vi "Convert FCS to PT3.vi"() -> ()   [LabVIEW 2012]
uses:
  Online acquisition/Online correlation/TTTR_data_headers/BINHDR_P.ctl
  Online acquisition/Online correlation/TTTR_data_headers/BOARDHDR.ctl
  Online acquisition/Online correlation/TTTR_data_headers/RtChan.ctl
  Online acquisition/Online correlation/TTTR_data_headers/TTTRHDR_P.ctl
  Online acquisition/Online correlation/TTTR_data_headers/TXTHDR.ctl
panel:
  out "Progress":dbl(slide) scale=0.0..100.0
  in  "Tab PH300":enum32{"PicoHarp 300 pt3 headers"}(tab)
  out "BINHDR_P":T1
  out "BOARDHDR":T2={"HardwareIdent[16]"="PicoHarp 300", "HardwareVersion[8]"="2.0", "HardwareSerial"=1006456, "SyncDivider"=8, "CFDZeroCross0"=10, "CFDLevel0"=200, "CFDZeroCross1"=10, "CFDLevel1"=200, "Resolution"=0.016, "RouterModelCode"=0, "RouterEnabled"=1, "RtChan"=[{"InputType"=1, "InputLevel"=-325, "InputEdge"=0, "CFDPresent"=0, "CFDLevel"=0, "CFDZeroCross"=0}, {"InputType"=1, "InputLevel"=-325, "InputEdge"=0, "CFDPresent"=0, "CFDLevel"=0, "CFDZeroCross"=0}, {"InputType"=2, "InputLevel"=760, "InputEdge"=1, "CFDPresent"=0, "CFDLevel"=1, "CFDZeroCross"=0}, {"InputType"=2, "InputLevel"=760, "InputEdge"=1, "CFDPresent"=0, "CFDLevel"=1, "CFDZeroCross"=0}]}
  out "TTTRHDR_P":T4={"ExtDevices"=0, "Reserved1"=0, "Reserved2"=0, "CntRate0"=79742000, "CntRate1"=420, "StopAfter"=40064, "StopReason"=1, "Records"=1168491, "ImgHdrSize"=0}
  out "TXTHDR":T5
  out "TTTR File":path=path "C:/Data Temporary/120823_PY3304testing/calibration30.pt3"
  out "Headers":T6(array[cluster])
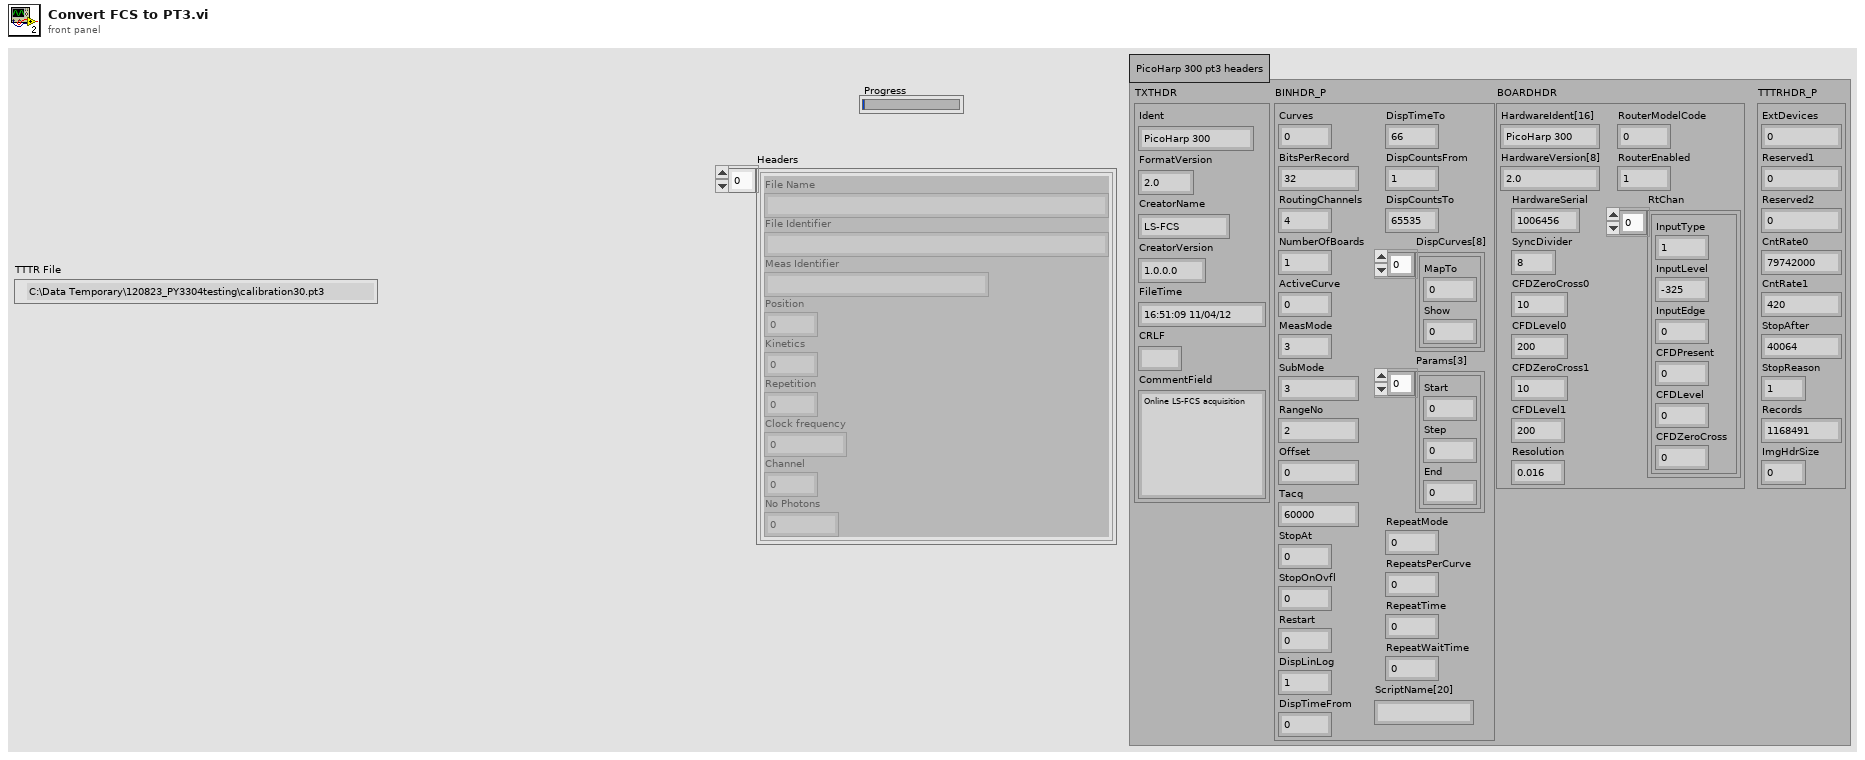
[diagram p1: front panel]
types:
  T1 = typedef "BINHDR_P.ctl" = cluster{"Curves":i32, "BitsPerRecord":i32, "RoutingChannels":i32, "NumberOfBoards":i32, "ActiveCurve":i32, "MeasMode":i32, "SubMode":i32, "RangeNo":i32, "Offset":i32, "Tacq":i32, "StopAt":i32, "StopOnOvfl":i32, "Restart":i32, "DispLinLog":i32, "DispTimeFrom":i32, "DispTimeTo":i32, "DispCountsFrom":i32, "DispCountsTo":i32, "DispCurves[8]":cluster{"MapTo":i32, "Show":i32}[], "Params[3]":cluster{"Start":sgl, "Step":sgl, "End":sgl}[], "RepeatMode":i32, "RepeatsPerCurve":i32, "RepeatTime":i32, "RepeatWaitTime":i32, "ScriptName[20]":string}
  T2 = typedef "BOARDHDR.ctl" = cluster{"HardwareIdent[16]":string, "HardwareVersion[8]":string, "HardwareSerial":i32, "SyncDivider":i32, "CFDZeroCross0":i32, "CFDLevel0":i32, "CFDZeroCross1":i32, "CFDLevel1":i32, "Resolution":sgl, "RouterModelCode":i32, "RouterEnabled":i32, "RtChan":T3}
  T3 = typedef "RtChan.ctl" = cluster{"InputType":i32, "InputLevel":i32, "InputEdge":i32, "CFDPresent":i32, "CFDLevel":i32, "CFDZeroCross":i32}[]
  T4 = typedef "TTTRHDR_P.ctl" = cluster{"ExtDevices":i32, "Reserved1":i32, "Reserved2":i32, "CntRate0":i32, "CntRate1":i32, "StopAfter":i32, "StopReason":i32, "Records":u32, "ImgHdrSize":i32}
  T5 = typedef "TXTHDR.ctl" = cluster{"Ident":string, "FormatVersion":string, "CreatorName":string, "CreatorVersion":string, "FileTime":string, "CRLF":string, "CommentField":string}
  T6 = cluster{"File Name":string, "File Identifier":string, "Meas Identifier":string, "Position":u32, "Kinetics":u32, "Repetition":u32, "Clock frequency":u32, "Channel":i32, "No Photons":i32}[]
  T7 = enum16{"big-endian, network order", "native, host order", "little-endian"}
  T8 = enum16{"open", "replace", "create", "open or create", "replace or create", "replace or create with confirmation"}
  T9 = cluster{"File Name":string, "File Identifier":string, "Meas Identifier":string, "Position":u32, "Kinetics":u32, "Repetition":u32, "Clock frequency":u32, "Channel":i32, "No Photons":i32}
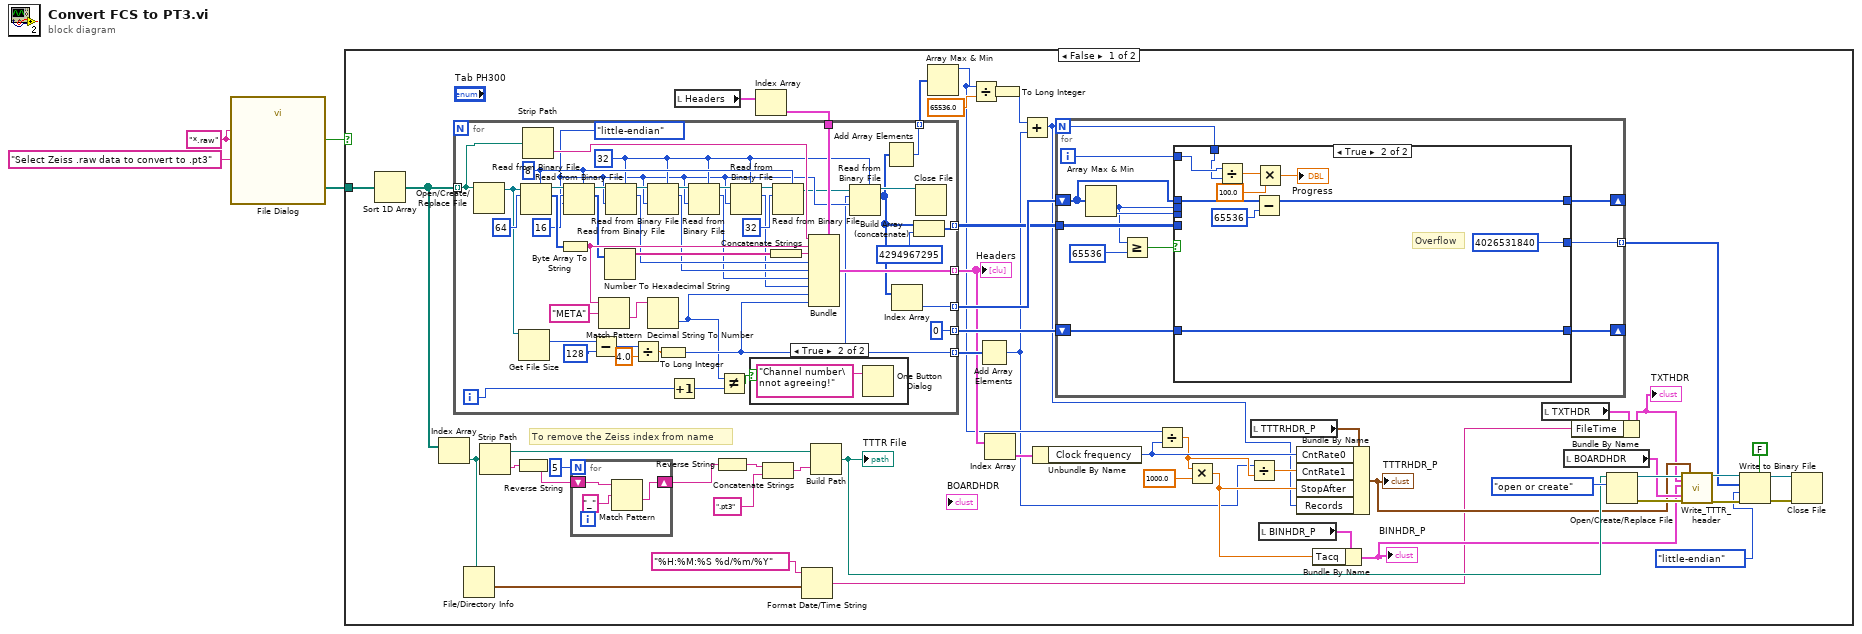
[diagram p0: block diagram]
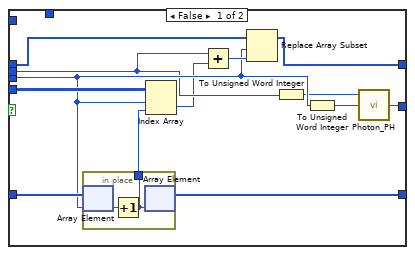
[diagram p2: hidden frame]
diagram:
  w3 = "*.raw" ("pattern label")
  n1 = call "File Dialog"("prompt"="Select Zeiss .raw data to convert to .pt3", "pattern (all files)"=w3, "pattern label"=w3) -> ("selected paths"=w1:path[], "cancelled"=w2:bool)  [unwired: 9 in, 2 out]
  n2 = case shown="False" w2 {
    tunnel: w1 -> [w12 _]
    frame False {
      # "To remove the Zeiss index from name"
      n3 = Sort 1D Array(array=w12) -> (sorted array=w11:path[])
      n4 = Index Array(array=w11) -> (element=w9:path)  [unwired: 1 in]
      n5 = File/Directory Info(path=w9) -> (last mod=w8:timestamp)  [unwired: 1 in, 6 out]
      n6 = Strip Path(path=w9) -> (stripped path=w46:path, name=w48:string)
      n7 = Reverse String(1:w48) -> (0:w16:string)
      n8 = for {
        N: 5 -> [_]
        shift-right: [w57] -> w15
        shift-left: w16 -> [w58]
        n9 = Match Pattern(string=w58, regular expression="_") -> (after substring=w57:string)  [unwired: 1 in, 3 out]
      }
      n10 = local read "Headers"() -> (w56:T6)
      n11 = Reverse String(1:w15) -> (0:w14:string)
      n12 = Index Array(array=w56) -> (element=w55:T9)  [unwired: 1 in]
      n13 = for {
        tunnel: w11 -> [w126] mode=indexing
        tunnel: [w127] -> w42 mode=indexing
        tunnel: w55 -> [w131]
        tunnel: [w104] -> w23 mode=indexing
        tunnel: [w108] -> w54 mode=indexing
        tunnel: [w103] -> w53 mode=indexing
        tunnel: [0 ("y")] -> w52 mode=indexing
        tunnel: [w101] -> w19 mode=indexing
        i -> [w100]
        w120 = T7."little-endian" ("byte order (0:big-endian, network order)")
        w121 = u32 32 ("count (1)")
        w132 = u8 8 ("count (1)")
        n14 = Open/Create/Replace File(file path (use dialog)=w126) -> (refnum out=w113:refnum<file>)  [unwired: 5 in, 2 out]
        n15 = Get File Size(file=w113) -> (size (in bytes)=w114:i64)  [unwired: 1 in, 2 out]
        n16 = Read from Binary File(5:w132, 10:64 ("count (1)"), 11:w113) -> (2:w141:u8[], 3:w140:refnum<file>)  [unwired: 3 in, 2 out]
        n17 = Strip Path(path=w126) -> (name=w125:string)  [unwired: 1 out]
        n18 = Byte Array To String(unsigned byte array=w141) -> (string=w130:string)
        n19 = Read from Binary File(5:w132, 9:w120, 10:16 ("count (1)"), 11:w140) -> (2:w122:u8[], 3:w139:refnum<file>)  [unwired: 2 in, 2 out]
        n20 = Subtract(x=w114, y=i64 128) -> (x-y=w112:i64)
        n21 = Match Pattern(string=w130, regular expression="META") -> (after substring=w128:string)  [unwired: 1 in, 3 out]
        n22 = Number To Hexadecimal String(2:w122) -> (0:w124:string[])  [unwired: 1 in]
        n23 = Read from Binary File(5:w121, 9:w120, 11:w139) -> (2:w119:u32, 3:w138:refnum<file>)  [unwired: 3 in, 2 out]
        n24 = Divide(x=w112, y=4.0) -> (x/y=w109:dbl)
        n25 = Read from Binary File(5:w121, 9:w120, 11:w138) -> (2:w118:u32, 3:w136:refnum<file>)  [unwired: 3 in, 2 out]
        n26 = Decimal String To Number(string=w128) -> (number=w98:i32)  [unwired: 2 in, 1 out]
        n27 = To Long Integer(number=w109) -> (32bit integer=w108:i32)
        n28 = Increment(x=w100) -> (x+1=w99:i32)
        n29 = Read from Binary File(5:w121, 9:w120, 11:w136) -> (2:w117:u32, 3:w135:refnum<file>)  [unwired: 3 in, 2 out]
        n30 = Not Equal?(x=w98, y=w99) -> (x != y?=w97:bool)
        n31 = Read from Binary File(5:w121, 9:w120, 11:w135) -> (2:w116:u32, 3:w134:refnum<file>)  [unwired: 3 in, 2 out]
        n32 = case shown="True" w97 {
          frame False {
          }
          frame True {
            n33 = One Button Dialog(message="Channel number\nnot agreeing!") -> ()  [unwired: 1 in, 1 out]
          }
        }
        n34 = Concatenate Strings(w124) -> (w123:string)
        n35 = Read from Binary File(5:w132, 10:32 ("count (1)"), 11:w134) -> (3:w115:refnum<file>)  [unwired: 3 in, 3 out]
        n36 = Bundle(cluster=w131, "File Name"=w125, "File Identifier"=w130, "Meas Identifier"=w123, "Position"=w119, "Kinetics"=w118, "Repetition"=w117, "Clock frequency"=w116, "Channel"=w98, "No Photons"=w108) -> (w127:T9)
        n37 = Read from Binary File(5:w121, 9:w120, 10:w108, 11:w115) -> (2:w102:u32[], 3:w107:refnum<file>)  [unwired: 2 in, 2 out]
        n38 = Add Array Elements(numeric array=w102) -> (sum=w101:u32)
        n39 = Index Array(array=w102) -> (element=w103:u32)  [unwired: 1 in]
        n40 = Build Array (concatenate)(w102, u32 4294967295 ("count (1)")) -> (w104:u32[])
        n41 = Close File(refnum=w107) -> ()  [unwired: 1 in, 2 out]
      }
      "Headers" <- w42
      n42 = Concatenate Strings(w14, ".pt3" ("regular expression")) -> (w45:string)
      n43 = Format Date/Time String(time format string (%c)="%H:%M:%S %d/%m/%Y", seconds (now)=w8) -> (date/time string=w7:string)  [unwired: 1 in]
      n44 = Build Path(base path=w46, name or relative path=w45) -> (appended path=w44:path)
      "TTTR File" <- w44
      n45 = Array Max & Min(array=w19) -> (max value=w20:u32)  [unwired: 3 out]
      n46 = Divide(x=w20, y=65536.0) -> (x/y=w21:dbl)
      n47 = Add Array Elements(numeric array=w54) -> (sum=w18:i32)
      n48 = Index Array(array=w42) -> (element=w41:T9)  [unwired: 1 in]
      n49 = To Long Integer(number=w21) -> (32bit integer=w10:i32)
      n50 = Add(x=w10, y=w18) -> (x+y=w17:i32)
      n51 = Unbundle By Name(w41) -> ("Clock frequency"=w40:u32)
      n52 = for {
        N: w17 -> [w60]
        shift-right: [w70] -> _
        shift-left: w53 -> [w71]
        tunnel: w23 -> [w69]
        shift-right: [w67] -> _
        shift-left: w52 -> [w68]
        tunnel: [w64] -> w24 mode=indexing
        i -> [w61]
        n53 = Array Max & Min(array=w71) -> (min value=w65:u32, min index (indices)=w66:i32)  [unwired: 2 out]
        n54 = Greater Or Equal?(x=w65, y=u32 65536) -> (x >= y?=w63:bool)
        n55 = case shown="True" w63 {
          tunnel: w71 -> [w84 w95]
          tunnel: [w82 w93] -> w70
          tunnel: w69 -> [w81 _]
          tunnel: w68 -> [w80 w94]
          tunnel: [w79 w94] -> w67
          tunnel: w66 -> [w76 _]
          tunnel: w65 -> [w74 _]
          tunnel: [w77 u32 4026531840 ("Event")] -> w64
          tunnel: w61 -> [_ w91]
          tunnel: w60 -> [_ w90]
          frame False {
            n56 = in-place {
              in-place-border: [w85] -> w78
              n57 = in-place-array #1(w80, w76) -> (w86:i32)
              n58 = Increment(x=w86) -> (x+1=w85:i32)
              n59 = in-place-array #1(w85) -> (w79:i32[])  [unwired: 1 out]
            }
            n60 = Index Array(array=w81, index (row)=w76, index (col)=w78) -> (element=w73:u32)
            n61 = Add(x=w74, y=w73) -> (x+y=w83:u32)
            n62 = Replace Array Subset(array=w84, new element=w83, index=w76) -> (w82:u32[])
            n63 = To Unsigned Word Integer(number=w74) -> (unsigned 16bit integer=w72:u16)
            n64 = To Unsigned Word Integer(number=w76) -> (unsigned 16bit integer=w75:u16)
            n65 = call "Photon_PH.vi"("dtime"=w75, "numsync"=w72) -> ("Event"=w77:u32)  [unwired: 1 in]
          }
          frame True {
            # "Overflow"
            n66 = Divide(x=w91, y=w90) -> (x/y=w89:dbl)
            n67 = Subtract(x=w95, y=u32 65536) -> (x-y=w93:u32[])
            n68 = Multiply(x=w89, y=100.0) -> (x*y=→"Progress":dbl)
          }
        }
      }
      n69 = Divide(x=w20, y=w40) -> (x/y=w38:dbl)
      n70 = Multiply(x=w38, y=1000.0) -> (x*y=w35:dbl)
      n71 = Divide(x=w18, y=w38) -> (x/y=w37:dbl)
      n72 = local read "TTTRHDR_P"() -> (w43:T4)
      n73 = local read "BINHDR_P"() -> (w36:T1)
      n74 = Bundle By Name(cluster=w43, "CntRate0"=w40, "CntRate1"=w37, "StopAfter"=w35, "Records"=w17) -> (w31:T4)
      "TTTRHDR_P" <- w31
      n75 = Bundle By Name(cluster=w36, "Tacq"=w35) -> (w33:T1)
      "BINHDR_P" <- w33
      n76 = local read "TXTHDR"() -> (w32:T5)
      n77 = local read "BOARDHDR"() -> (w34:T2)
      n78 = Bundle By Name(cluster=w32, "FileTime"=w7) -> (w5:T5)
      "TXTHDR" <- w5
      n79 = Open/Create/Replace File(file path (use dialog)=w44, operation (0:open)=T8."open or create") -> (refnum out=w50:refnum<file>, error out=w51:errorcluster)  [unwired: 4 in, 1 out]
      n80 = call "Write_TTTR_header.vi"("TTTR Ref In"=w50, "TXTHDR"=w5, "BINHDR_P"=w33, "BOARDHDR"=w34, "Error In"=w51, "TTTRHDR_P"=w31) -> ("TTTR Ref Out"=w29:refnum<file>, "Error Out"=w30:errorcluster)  [unwired: 12 in]
      n81 = Write to Binary File(file (use dialog)=w29, data=w24, error in=w30, 5:FALSE ("prepend array or string size? (T)"), 9:T7."little-endian" ("byte order (0:big-endian, network order)")) -> (refnum out=w25:refnum<file>, error out=w26:errorcluster)  [unwired: 1 in, 1 out]
      n82 = Close File(refnum=w25, error in=w26) -> ()  [unwired: 2 out]
    }
    frame True {
    }
  }
